vi "Speed-Length_calculator.vi"(0 "Sensors_Distance [mm]":dbl, 1 "TriggerS1":bool, 2 "TriggerS2":bool, 3 "Max_Time [s]":dbl) -> (4 "Flag_EndMeasure":bool, 5 "Speed [mm/s]":dbl, 6 "Length [mm]":dbl, 7 "Alarm":bool)   [LabVIEW 2020]
doc: "From Rise/Fall edges of sensors calculate speed and length of piece and set alarm in case of stuck."
panel:
  out "Stop_T2 [s]":dbl format="%.20g"
  out "Start_T2 [s]":dbl format="%.20g"
  out "Stop_T1 [s]":dbl format="%.20g"
  out "Start_T1 [s]":dbl format="%.20g"
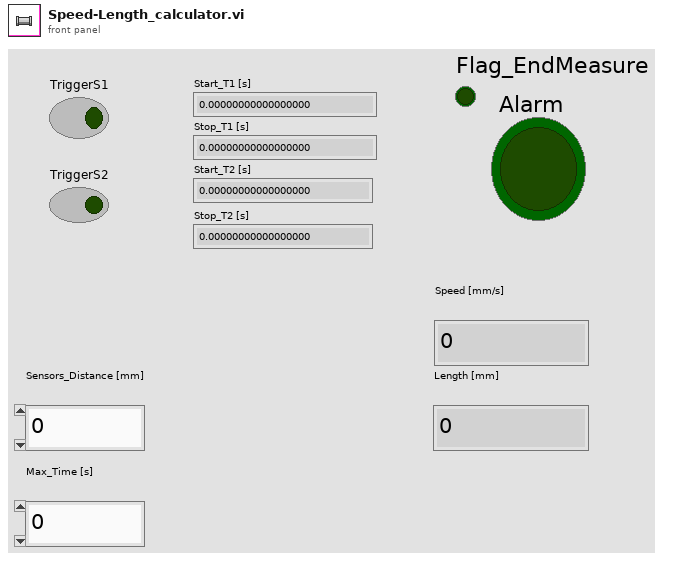
[diagram p1: front panel]
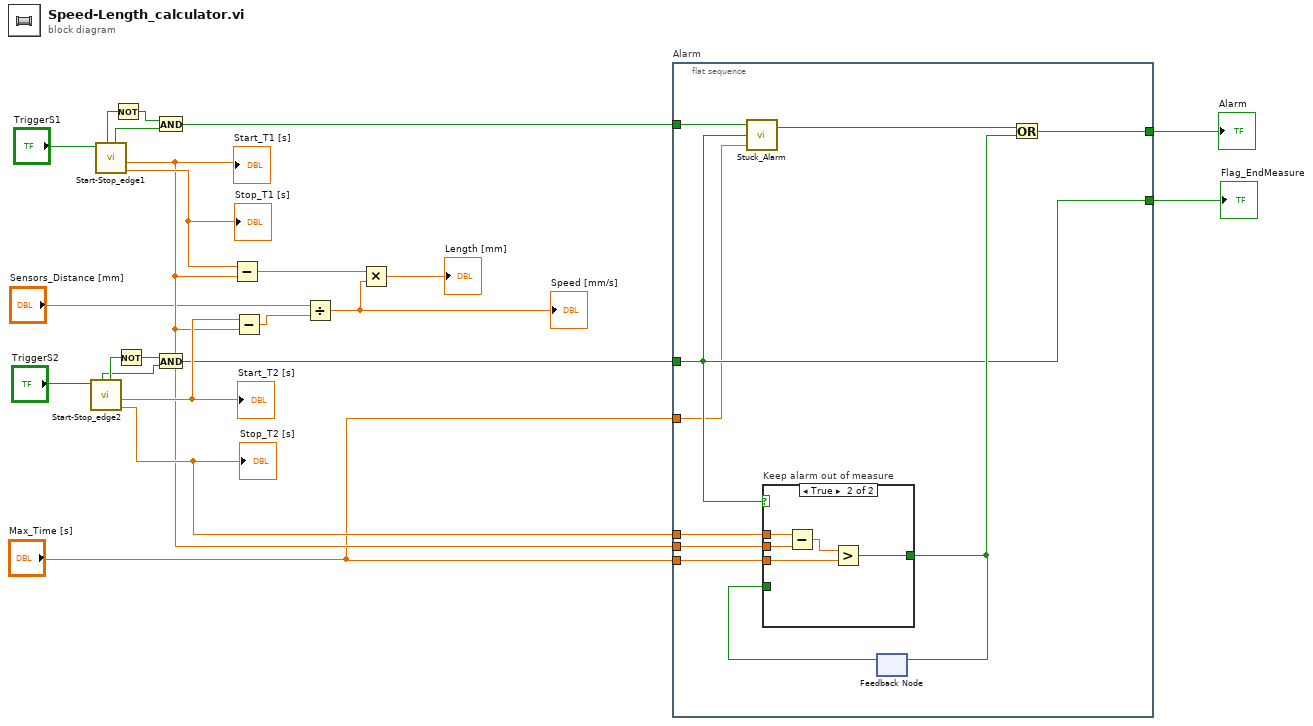
[diagram p0: block diagram]
diagram:
  n1 = call "Start-Stop_edge2.vi"("TriggerSn"="TriggerS2") -> ("Stop_Tn [s]"=w6:dbl, "Start_Tn [s]"=w18:dbl, "TriggerSn_prev0"=w13:bool, "TriggerSn_prev-1"=w12:bool)  [unwired: 7 in]
  "Start_T2 [s]" <- w18
  "Stop_T2 [s]" <- w6
  n2 = call "Start-Stop_edge1.vi"("TriggerSn"="TriggerS1") -> ("Stop_Tn [s]"=w20:dbl, "Start_Tn [s]"=w5:dbl, "TriggerSn_prev0"=w9:bool, "TriggerSn_prev-1"=w11:bool)  [unwired: 7 in]
  "Start_T1 [s]" <- w5
  "Stop_T1 [s]" <- w20
  n3 = Not(x=w11) -> (.not. x?=w10:bool)
  n4 = Not(x=w13) -> (.not. x?=w14:bool)
  n5 = And(x=w10, y=w9) -> (x .and. y?=w8:bool)
  n6 = And(x=w14, y=w12) -> (x .and. y?=w7:bool)
  n7 = Subtract(x=w20, y=w5) -> (x-y=w19:dbl)
  n8 = Subtract(x=w18, y=w5) -> (x-y=w17:dbl)
  n9 = Divide(x="Sensors_Distance [mm]", y=w17) -> (x/y=w16:dbl)
  "Speed [mm/s]" <- w16
  n10 = Multiply(x=w19, y=w16) -> (x*y=→"Length [mm]":dbl)
  n11 = flat-sequence "Alarm" {
    tunnel: w8 -> [w26]
    tunnel: w7 -> [w25]
    tunnel: "Max_Time [s]" -> [w24]
    tunnel: w6 -> [w32]
    tunnel: w5 -> [w31]
    tunnel: [w28] -> w4
    tunnel: [w25] -> w3
    tunnel: "Max_Time [s]" -> [w23]
    frame #0 {
      n12 = call "Stuck_Alarm.vi"("Time Target (s)"=w24, "Finish_Measurement"=w25, "Start_Measurement"=w26) -> ("Stuck_Alarm"=w27:bool)
      n13 = feedback #1() -> (w30:bool)  [unwired: 1 in]
      n14 = case "Keep alarm out of measure" shown="True" w25 {
        tunnel: w32 -> [_ w38]
        tunnel: w31 -> [_ w37]
        tunnel: [w33 w35] -> w29
        tunnel: w30 -> [w33 _]
        tunnel: w23 -> [_ w34]
        frame False {
        }
        frame True {
          n15 = Subtract(x=w38, y=w37) -> (x-y=w36:dbl)
          n16 = Greater?(x=w36, y=w34) -> (0:w35:bool)
        }
      }
      n17 = feedback-in #1(w29) -> ()
      n18 = Or(x=w27, y=w29) -> (x .or. y?=w28:bool)
    }
  }
  "Alarm" <- w4
  "Flag_EndMeasure" <- w3
